vi "check data from plc.vi"(10 "Pressure Auto":bool=TRUE, 11 "DATA":string="\u001b@;\u001bG1;\u001bH0;\u001bI 342;\u001bJ 189;\u001bL000;\u001bO 25;\u001bM020;\u001bU7673    955    804        ;\u001bZ;\u001bG1;\u001bH0;\u001bI 345;\u001bJ 302;\u001bL000;\u001bO 25;\u001bM020;\u001bUA001019;\u001bZ;\u001bG1;\u001bH0;\u001bI 545;\u001bJ 298;\u001bL000;\u001bO 25;\u001bM020;\u001bU@MM/YY@;\u001bZ;\u001b!;") -> (1 "Pressure":string, 2 "Sr. NO.":string, 3 "ZF PART NO.":string)   [LabVIEW 2015]
panel:
  out "Array 2":string[](array[string])
  out "array 2":string[](array[string])
  out "Array":string[](array[string])
  out "array":string[](array[string])
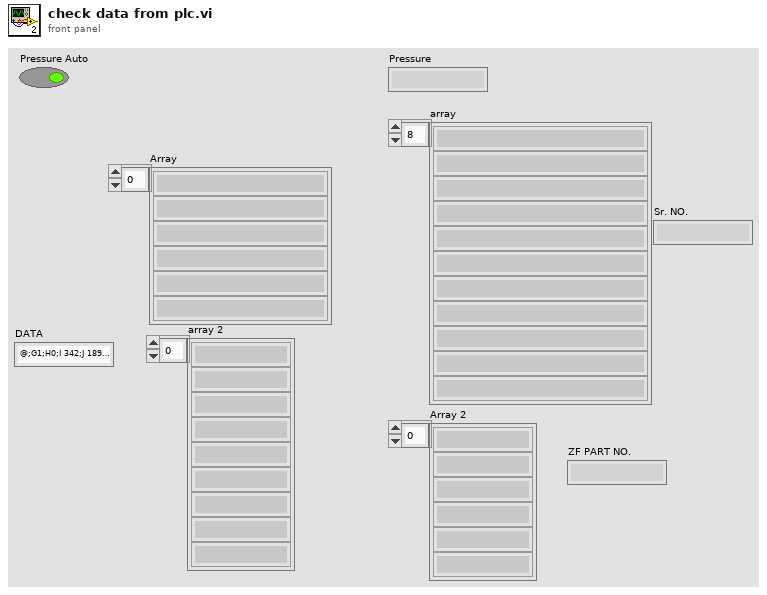
[diagram p1: front panel]
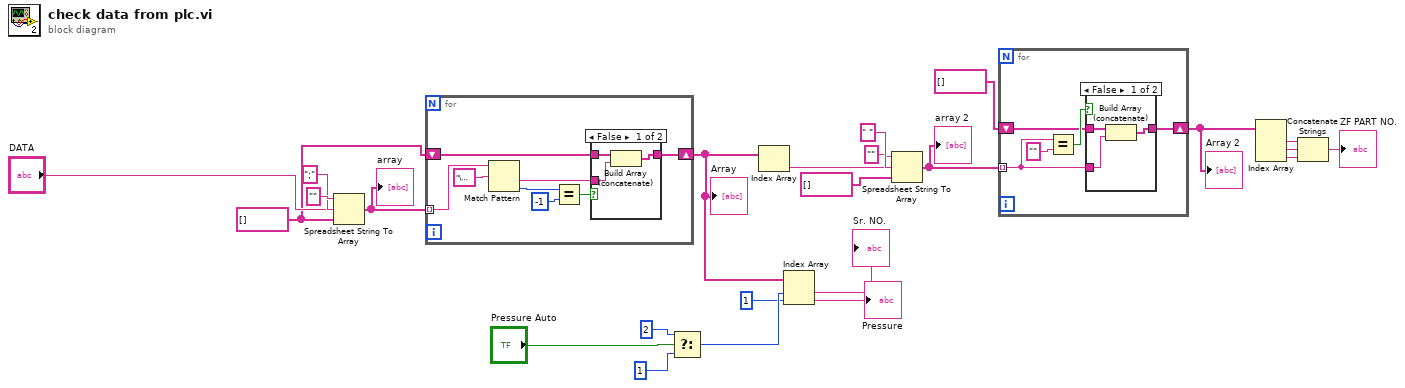
[diagram p0: block diagram]
diagram:
  w20 = string[] []
  n1 = Spreadsheet String To Array(delimiter (Tab)=";", format string="", spreadsheet string="DATA", array type (2D Dbl)=w20) -> (array=w21:string[])
  "array" <- w21
  n2 = for {
    tunnel: w21 -> [w32] mode=indexing
    shift-right: [w26] -> w8
    shift-left: w20 -> [w27]
    n3 = Match Pattern(string=w32, regular expression="\u001bU") -> (after substring=w25:string, offset past match=w30:i32)  [unwired: 1 in, 2 out]
    n4 = Equal?(x=w30, y=-1) -> (x = y?=w28:bool)
    n5 = case shown="False" w28 {
      tunnel: w27 -> [w35 w36]
      tunnel: [w34 w36] -> w26
      tunnel: w25 -> [w33 _]
      frame False {
        n6 = Build Array (concatenate)(w35, w33) -> (w34:string[])
      }
      frame True {
      }
    }
  }
  "Array" <- w8
  n7 = Select(t=2 ("index"), s="Pressure Auto", f=1 ("index")) -> (s? t:f=w3:i32)
  n8 = Index Array(array=w8) -> (element=w17:string)  [unwired: 1 in]
  n9 = Index Array(array=w8, index #1=w3, index #2=1 ("index")) -> (element #1=→"Sr. NO.":string, element #2=→"Pressure":string)
  n10 = Spreadsheet String To Array(delimiter (Tab)=" ", format string="", spreadsheet string=w17, array type (2D Dbl)=string[] []) -> (array=w14:string[])
  "array 2" <- w14
  n11 = for {
    tunnel: w14 -> [w37] mode=indexing
    shift-right: [w39] -> w13
    shift-left: string[] [] -> [w40]
    n12 = Equal?(x=w37, y="" ("regular expression")) -> (x = y?=w41:bool)
    n13 = case shown="False" w41 {
      tunnel: w40 -> [w44 w45]
      tunnel: [w43 w45] -> w39
      tunnel: w37 -> [w42 _]
      frame False {
        n14 = Build Array (concatenate)(w44, w42) -> (w43:string[])
      }
      frame True {
      }
    }
  }
  "Array 2" <- w13
  n15 = Index Array(array=w13) -> (element #1=w12:string, element #2=w11:string, element #3=w10:string)  [unwired: 3 in]
  n16 = Concatenate Strings(w12, w11, w10) -> (→"ZF PART NO.":string)
